vi "Init GUI Objects.vi"(8 "Error In":errorcluster, 9 "New Error":T1, 10 "Error Message":refnum<vi>, 11 "Error Code":refnum<vi>) -> (0 "Error Out":errorcluster)   [LabVIEW 2023, in "Error Manager.lvlib" / "New Error Window.lvlib"]
doc: "This VI configures the \"look and feel\" of GUI objects, and sets their value (their contents)."
uses:
  New Error Window.lvlib
  New Error (To Be Displayed To User) (cluster).ctl
  <vilib>/Utility/miscctls.llb/LVFontTypeDef.ctl
panel:
  # "Development\nControls or indicators that are useful for development or testing, but which are not outputs of the VI."
  # "Input\nInputs to the VI"
  # "Output\nOutputs of the VI"
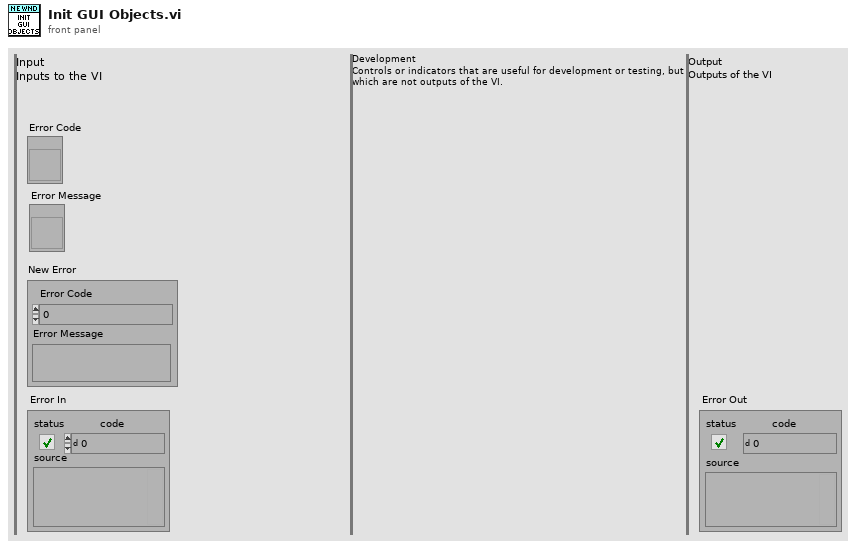
[diagram p1: front panel]
types:
  T1 = typedef "Error Manager.lvlib/New Error Window.lvlib/New Error (To Be Displayed To User) (cluster).ctl" = cluster{"Error Code":i32, "Error Message":string}
  T2 = typedef "LVFontTypeDef.ctl" = cluster{"Font Name":string, "Size":u16, "Bold":bool, "Italic":bool, "Underline":bool, "Strikeout":bool, "Color":u32}
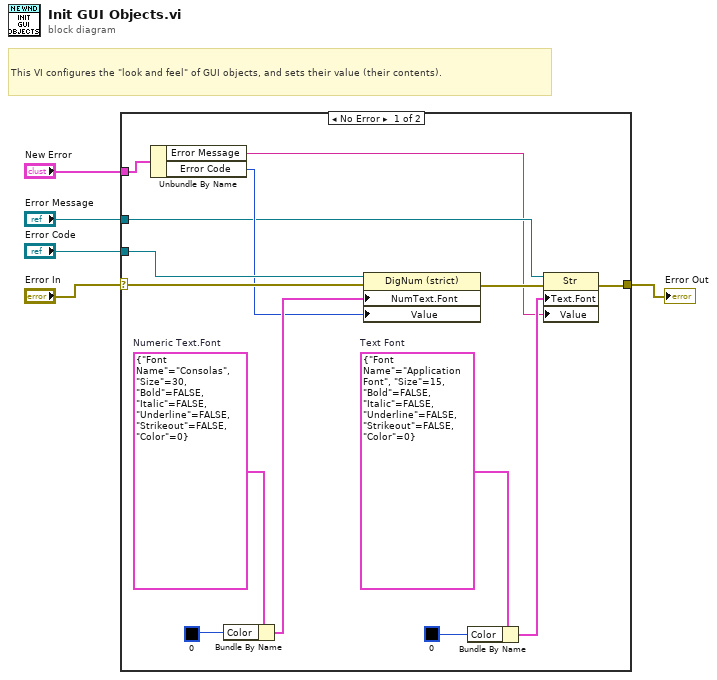
[diagram p0: block diagram]
diagram:
  # "This VI configures the \"look and feel\" of GUI objects, and sets their value (their contents)."
  n1 = case shown="No Error" "Error In" {
    selector: "Error In" -> [w19 w20]
    tunnel: [w10 w20] -> w4
    tunnel: "Error Code" -> [w18 _]
    tunnel: "Error Message" -> [w12 _]
    tunnel: "New Error" -> [w14 _]
    frame No Error {
      w9 = T2 {"Font Name"="Application Font", "Size"=15, "Bold"=FALSE, "Italic"=FALSE, "Underline"=FALSE, "Strikeout"=FALSE, "Color"=0}  # Text Font
      w17 = T2 {"Font Name"="Consolas", "Size"=30, "Bold"=FALSE, "Italic"=FALSE, "Underline"=FALSE, "Strikeout"=FALSE, "Color"=0}  # Numeric Text.Font
      n2 = Unbundle By Name(w14) -> ("Error Message"=w6:string, "Error Code"=w13:i32)
      n3 = Bundle By Name(cluster=w17, "Color"=u32 0) -> (w16:T2)
      n4 = property class="DigNum (strict)"(reference=w18, error in=w19, "NumText.Font"=w16, "Value"=w13) -> (error out=w11:errorcluster)  [unwired: 1 out]
      n5 = Bundle By Name(cluster=w9, "Color"=u32 0) -> (w8:T2)
      n6 = property class="Str"(reference=w12, error in=w11, "Text.Font"=w8, "Value"=w6) -> (error out=w10:errorcluster)  [unwired: 1 out]
    }
    frame Error {
    }
  }
  "Error Out" <- w4
